vi "MoveChuck.vi"() -> ()   [LabVIEW 2017]
uses:
  Interface.ctl
panel:
  in  "Y Pos":dbl=1000.0
  in  "X Pos":dbl=1000.0
  in  "Interface":T1
  in  "Absolution move?":bool
  out "error code":i32
  out "StringOutputArray":string[](array[string])
  out "Response":string
  in  "VISA Resource":refnum<visa-resource-name>="GPIB0::13::INSTR"
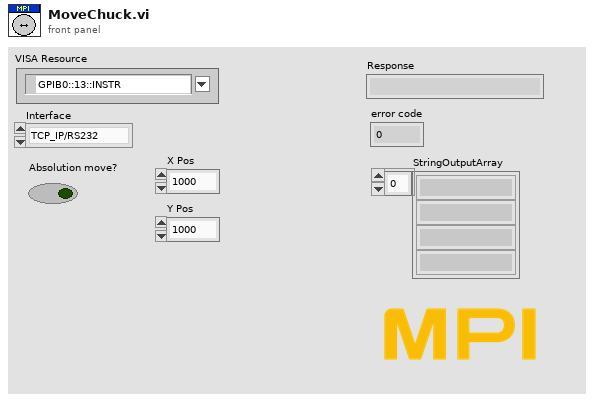
[diagram p1: front panel]
types:
  T1 = typedef "Interface.ctl" = enum16{"TCP_IP/RS232", "GPIB"}
  T2 = enum16{"EndOfLine", "LineFeed", "CarriageReturn"}
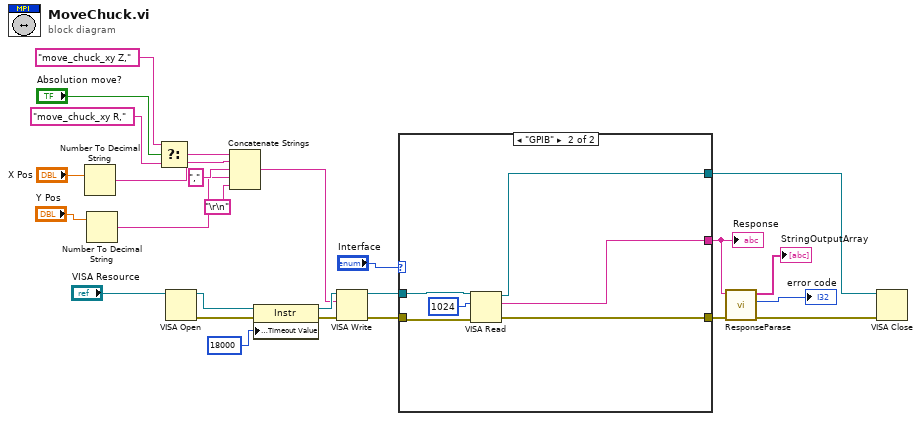
[diagram p0: block diagram]
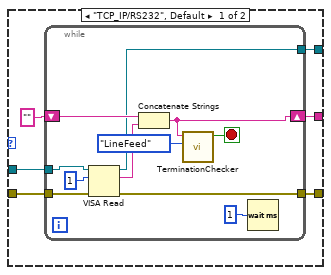
[diagram p2: hidden frame]
diagram:
  n1 = Number To Decimal String(number="X Pos") -> (decimal integer string=w6:string)  [unwired: 1 in]
  n2 = Number To Decimal String(number="Y Pos") -> (decimal integer string=w3:string)  [unwired: 1 in]
  n3 = Select(t="move_chuck_xy Z,", s="Absolution move?", f="move_chuck_xy R,") -> (s? t:f=w14:string)
  n4 = VISA Open(VISA resource name="VISA Resource") -> (VISA resource name=w24:refnum<visa-resource-name>, error out=w23:errorcluster)  [unwired: 1 in, 3 out]
  n5 = Concatenate Strings(w14, w6, ",", w3, "\r\n") -> (w20:string)
  n6 = property class="Instr"(reference=w24, error in=w23, "General Settings:Timeout Value"=u32 18000) -> (reference out=w22:refnum<visa-resource-name>, error out=w21:errorcluster)
  n7 = VISA Write(VISA resource name=w22, write buffer=w20, error in (no error)=w21) -> (VISA resource name out=w19:refnum<visa-resource-name>, error out=w18:errorcluster)  [unwired: 1 out]
  n8 = case shown="\"GPIB\"" "Interface" {
    tunnel: w19 -> [w32 w47]
    tunnel: w18 -> [w31 w48]
    tunnel: [w29 w44] -> w17
    tunnel: [w28 w46] -> w11
    tunnel: [w27 w45] -> w10
    frame "TCP_IP/RS232", Default {
      n9 = while {
        tunnel: w32 -> [w43]
        tunnel: w31 -> [w42]
        shift-right: [w36] -> w29
        shift-left: "" -> [w40]
        tunnel: [w34] -> w27
        tunnel: [w33] -> w28
        stop <- w38 stop-if-true
        n10 = VISA Read(VISA resource name=w43, byte count=u32 1, error in (no error)=w42) -> (VISA resource name out=w34:refnum<visa-resource-name>, read buffer=w39:string, error out=w33:errorcluster)  [unwired: 1 out]
        n11 = Concatenate Strings(w40, w39) -> (w36:string)
        n12 = call "TerminationChecker.vi"("Type"=T2."LineFeed", "input string"=w36) -> ("Ret"=w38:bool)  [unwired: 9 in]
        n13 = Wait (ms)(milliseconds to wait=u32 1) -> ()  [unwired: 1 out]
      }
    }
    frame "GPIB" {
      n14 = VISA Read(VISA resource name=w47, byte count=u32 1024, error in (no error)=w48) -> (VISA resource name out=w45:refnum<visa-resource-name>, read buffer=w44:string, error out=w46:errorcluster)  [unwired: 1 out]
    }
  }
  "Response" <- w17
  n15 = call "ResponseParase.vi"("error in (no error)"=w11, "input string"=w17) -> ("error out"=w1:errorcluster, "error code"=→"error code":i32, "OutputArray"=→"StringOutputArray":string[])  [unwired: 7 in]
  n16 = VISA Close(VISA resource name=w10, error in (no error)=w1) -> ()  [unwired: 1 out]
